vi "LimelightSeeker.vi"(9 "TargetDistance":dbl, 10 "TargetX":dbl) -> (1 "rightMotorSpeed":dbl, 2 "leftMotorSpeed":dbl)   [LabVIEW 2018]
panel:
  in  "kPDistAdj":dbl
  in  "StopDistance":dbl=24.0
  in  "Deadband":dbl=3.0
  in  "MinAimCommand":dbl=0.06
  in  "BaseSpeed":dbl=0.1
  in  "kPDrive":dbl=0.3
  in  "kPAim":dbl=0.01
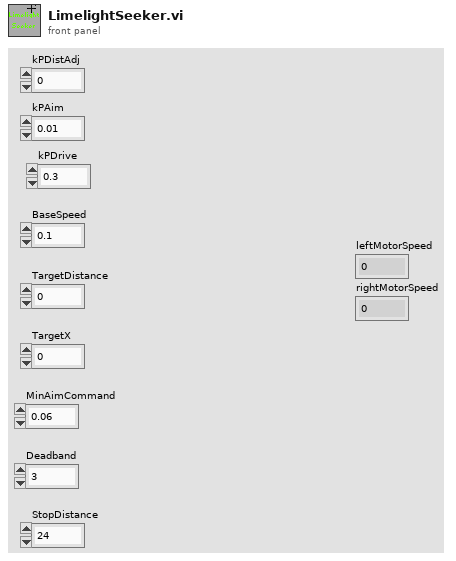
[diagram p1: front panel]
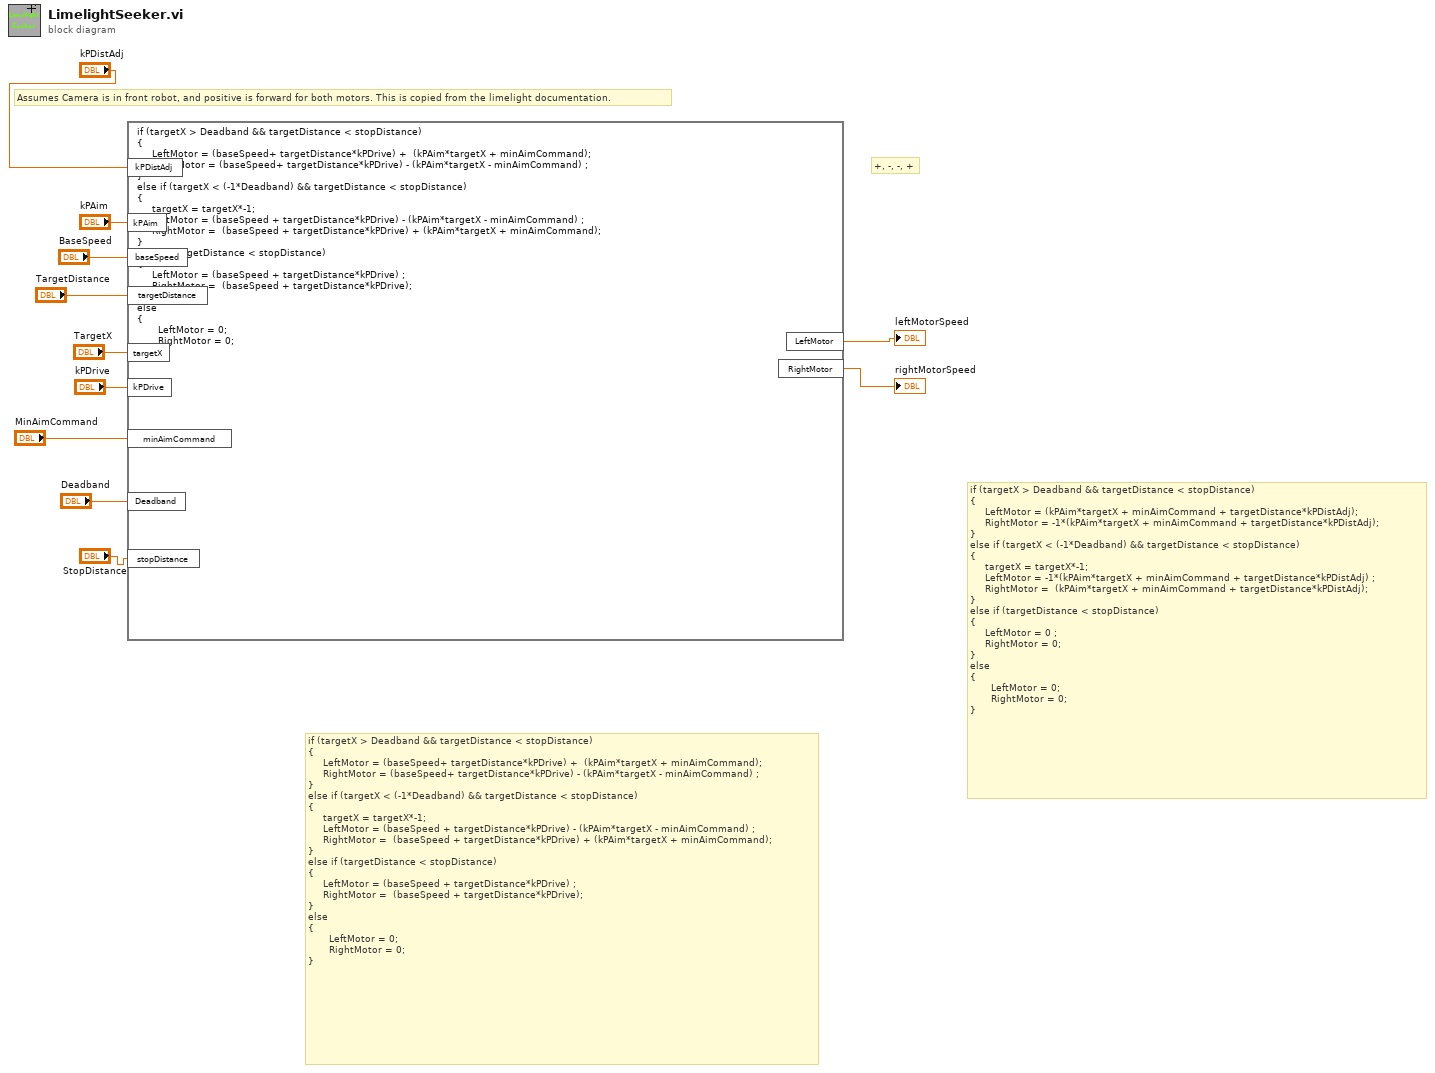
[diagram p0: block diagram]
diagram:
  # "if (targetX > Deadband && targetDistance < stopDistance) \n{\n     LeftMotor = (kPAim*targetX + minAimCommand + targetDistance*kPDistAdj); \n     RightMotor = -1*(kPAim*targetX + minAimCommand + targetDistance*kPDistAdj);\n}\nelse if (targetX < (-1*Deadband) && targetDistance < stopDistance)\n{\n     targetX = targetX*-1;\n     LeftMotor = -1*(kPAim*targetX + minAimCommand + targetDistance*kPDistAdj) ;\n     RightMotor =  (kPAim*targetX + minAimCommand + targetDistance*kPDistAdj);\n}\nelse if (targetDistance < stopDistance)\n{\n     LeftMotor = 0 ;\n     RightMotor = 0;\n}\nelse\n{\n       LeftMotor = 0;\n       RightMotor = 0;\n}"
  # "+, -, -, +"
  # "if (targetX > Deadband && targetDistance < stopDistance) \n{\n     LeftMotor = (baseSpeed+ targetDistance*kPDrive) +  (kPAim*targetX + minAimCommand);\n     RightMotor = (baseSpeed+ targetDistance*kPDrive) - (kPAim*targetX - minAimCommand) ;\n}\nelse if (targetX < (-1*Deadband) && targetDistance < stopDistance)\n{\n     targetX = targetX*-1;\n     LeftMotor = (baseSpeed + targetDistance*kPDrive) - (kPAim*targetX - minAimCommand) ;\n     RightMotor =  (baseSpeed + targetDistance*kPDrive) + (kPAim*targetX + minAimCommand);\n}\nelse if (targetDistance < stopDistance)\n{\n     LeftMotor = (baseSpeed + targetDistance*kPDrive) ;\n     RightMotor =  (baseSpeed + targetDistance*kPDrive);\n}\nelse\n{\n       LeftMotor = 0;\n       RightMotor = 0;\n}"
  # "Assumes Camera is in front robot, and positive is forward for both motors. This is copied from the limelight documentation."
  n1 = formula code="if (targetX > Deadband && targetDistance < stopDistance) \n{\n     LeftMotor = (baseSpeed+ targetDistance*kPDrive) +  (kPAim*targetX + minAimCommand);\n     RightMotor = (baseSpeed+ targetDistance*kPDrive) - (kPAim*targetX - minAimCommand) ;\n}\nelse if (targetX < (-1*Deadband) && targetDistance < stopDistance)\n{\n     targetX = targetX*-1;\n     LeftMotor = (baseSpeed + targetDistance*kPDrive) - (kPAim*targetX - minAimCommand) ;\n     RightMotor =  (baseSpeed + targetDistance*kPDrive) + (kPAim*targetX + minAimCommand);\n}\nelse if (targetDistance < stopDistance)\n{\n     LeftMotor = (baseSpeed + targetDistance*kPDrive) ;\n     RightMotor =  (baseSpeed + targetDistance*kPDrive);\n}\nelse\n{\n       LeftMotor = 0;\n       RightMotor = 0;\n}"("kPAim"="kPAim", "baseSpeed"="BaseSpeed", "targetDistance"="TargetDistance", "targetX"="TargetX", "kPDrive"="kPDrive", "minAimCommand"="MinAimCommand", "Deadband"="Deadband", "stopDistance"="StopDistance", "kPDistAdj"="kPDistAdj") -> ("LeftMotor"=→"leftMotorSpeed":dbl, "RightMotor"=→"rightMotorSpeed":dbl)
